vi "Request Synchronous Timestamp.vi"(6 "Ignore Past Updates? (F)":bool, 7 "Timeout In ms (-1)":i32=-1, 8 "error in (no error)":errorcluster, 9 "Type (Timestamp)":timestamp, 10 "Datum Name":string, 11 "IObserver In":refnum<class "IObserver.lvclass">) -> (0 "error out":errorcluster, 1 "timed out?":bool, 2 "Data (Timestamp)":timestamp, 4 "Publication Time":timestamp)   [LabVIEW 2018, in "MVA Framework.lvlib" / "IObserver.lvlib" / "IObserver.lvclass"]
doc: "此 VI 已过时，请使用 Request Synchronous Data.vim"
uses:
  IObserver.lvclass
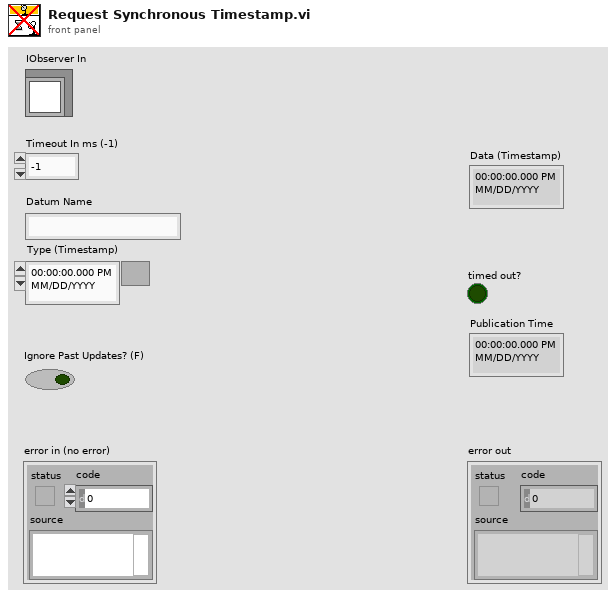
[diagram p1: front panel]
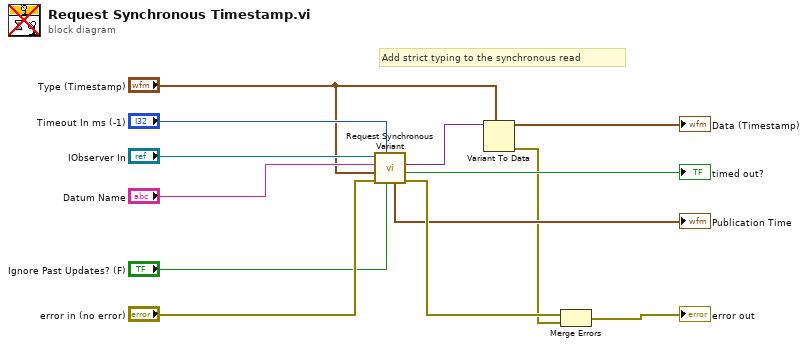
[diagram p0: block diagram]
diagram:
  # "Add strict typing to the synchronous read"
  n1 = call "Request Synchronous Variant.vi"("Ignore Past Updates? (F)"="Ignore Past Updates? (F)", "Timeout In ms (-1)"="Timeout In ms (-1)", "error in (no error)"="error in (no error)", "Type"="Type (Timestamp)", "Datum Name"="Datum Name", "IObserver In"="IObserver In") -> ("error out"=w10:errorcluster, "timed out?"=→"timed out?":bool, "Data"=w6:variant, "Publication Time"=→"Publication Time":timestamp)  [unwired: 2 in]
  n2 = Variant To Data(type="Type (Timestamp)", Variant=w6) -> (data=→"Data (Timestamp)":timestamp, error out=w1:errorcluster)  [unwired: 1 in]
  n3 = Merge Errors(w10, w1) -> (→"error out":errorcluster)
